vi "DCRI.vi"() -> ()   [LabVIEW 2024]
uses:
  EFmeter.lvlib
  <vilib>/Analysis/NI_AALBase.lvlib
  <vilib>/Analysis/baseanly.llb/Mean (DBL).vi
  BK Precision 8500B Series/BK Precision 8500B Series.lvlib
  <instrlib>/Zatez Kopper/Zatez Kopper.lvlib
panel:
  out "Aktualni zatez 2":dbl=2.5
  out "DCIR":dbl
  in  "Èas ustálení [ms]":dbl
  in  "LOAD":refnum<visa-resource-name>
  in  "Clear":bool
  in  "Typ zateze":u16(ring) items=["Manualni", "BK 8542B", "KOPPER-zatez"]
  in  "Ulozit data":bool
  in  "file path (use dialog)":path
  in  "Vzorku na krokù":u16 max=100 step=1
  in  "Prumerovani":bool
  in  "Zatezovaci proud [A]":dbl
  in  "EFmeter":refnum<visa-resource-name>
  in  "stop":bool
  in  "Start":bool
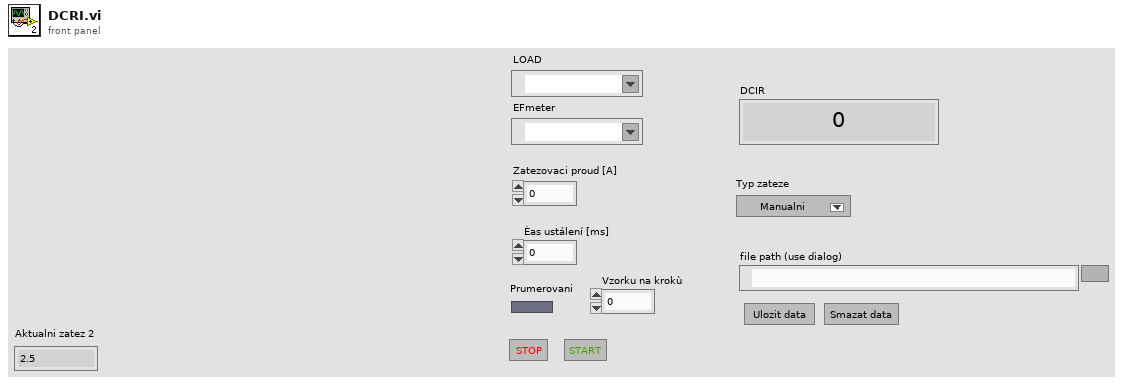
[diagram p1: front panel]
types:
  T1 = enum16{"init", "wait", "graph", "meas", "change_load", "init_measurment", "save", "clear"}
  T2 = enum16{"open", "replace", "create", "open or create", "replace or create", "replace or create with confirmation"}
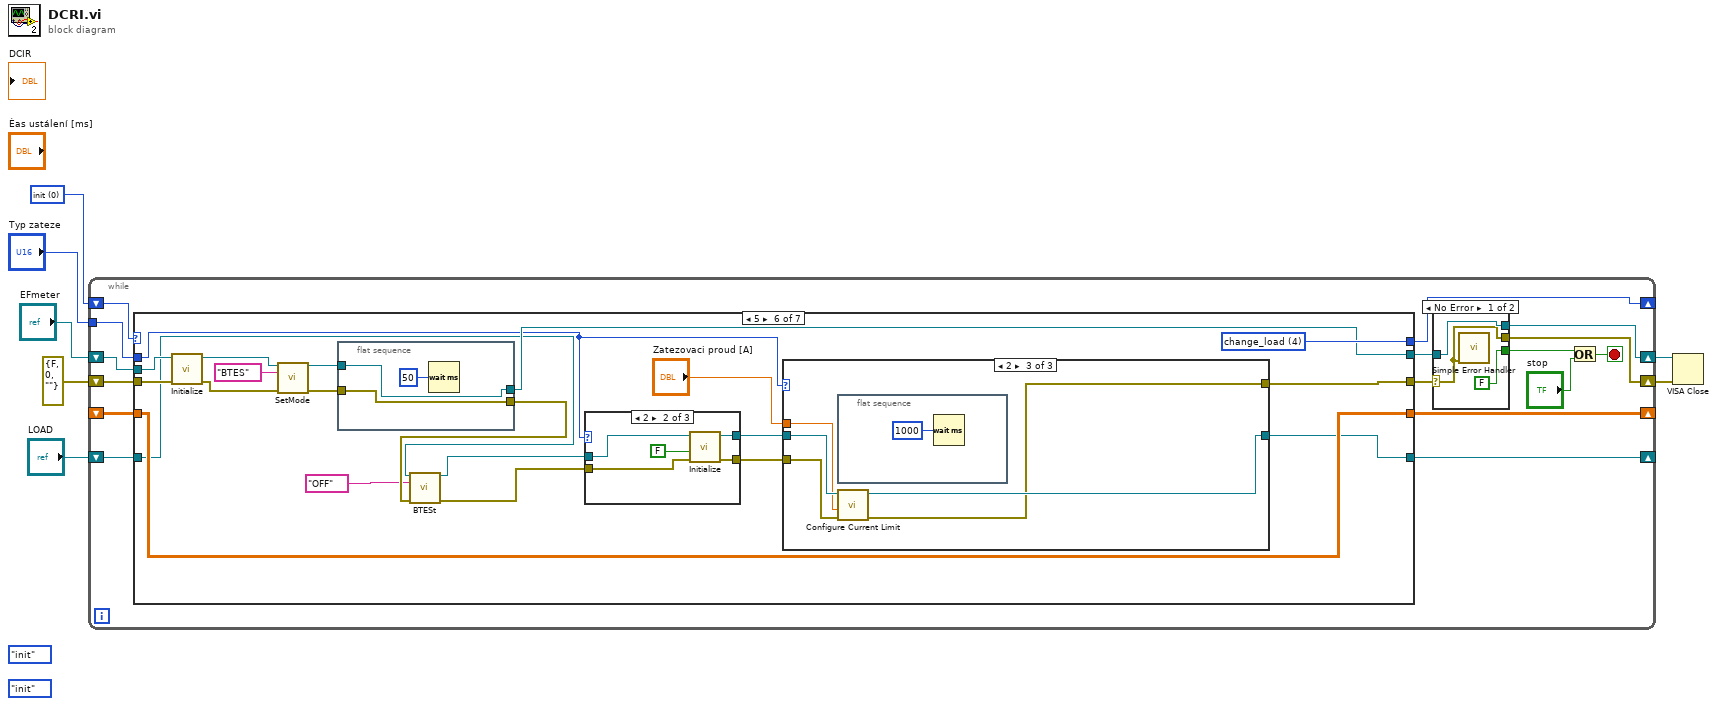
[diagram p0: block diagram]
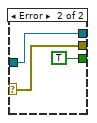
[diagram p2: hidden frame]
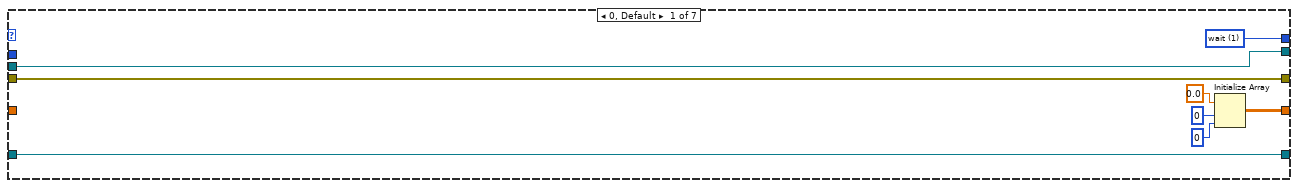
[diagram p3: hidden frame]
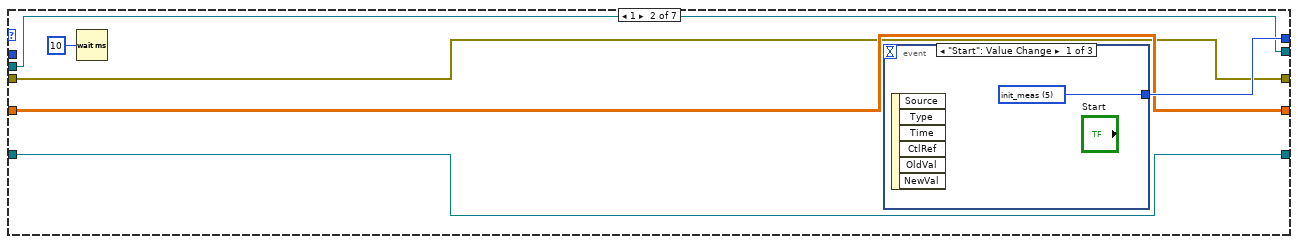
[diagram p4: hidden frame]
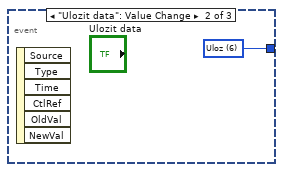
[diagram p5: hidden frame]
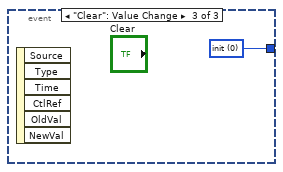
[diagram p6: hidden frame]
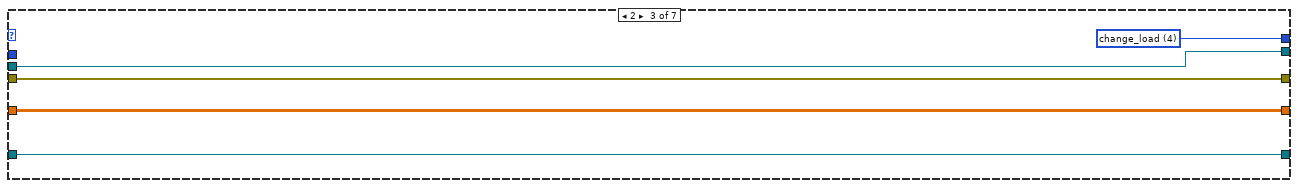
[diagram p7: hidden frame]
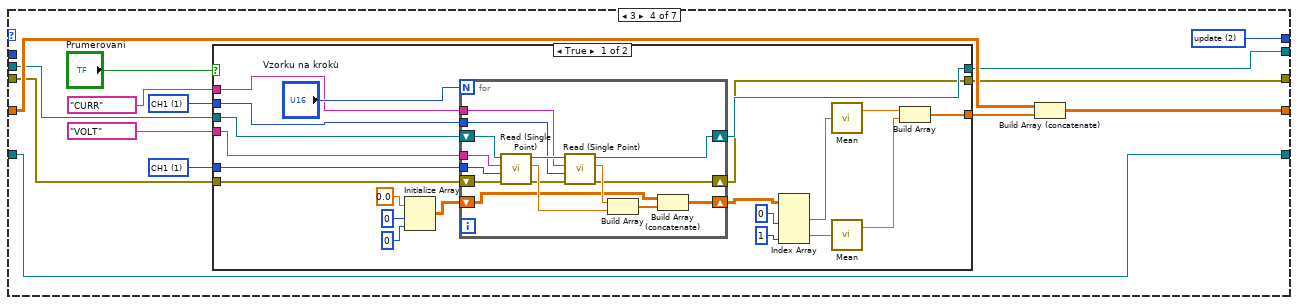
[diagram p8: hidden frame]
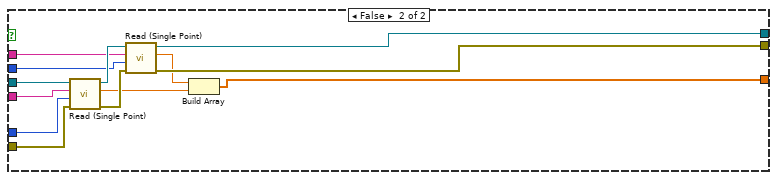
[diagram p9: hidden frame]
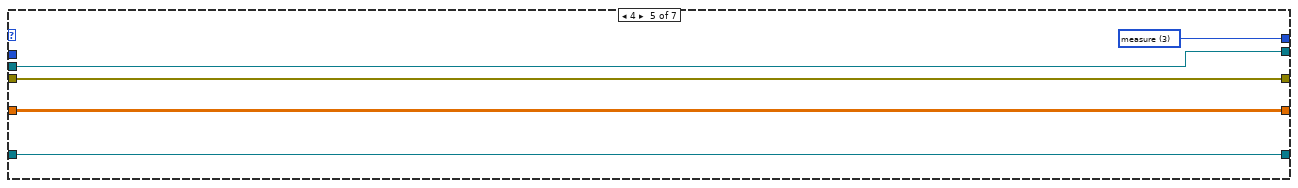
[diagram p10: hidden frame]
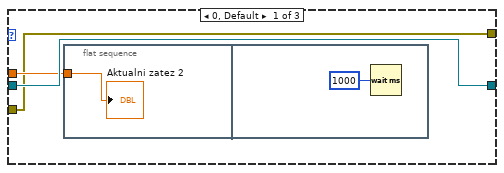
[diagram p11: hidden frame]
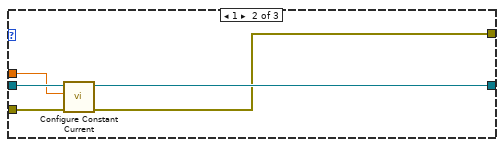
[diagram p12: hidden frame]
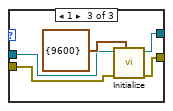
[diagram p14: hidden frame]
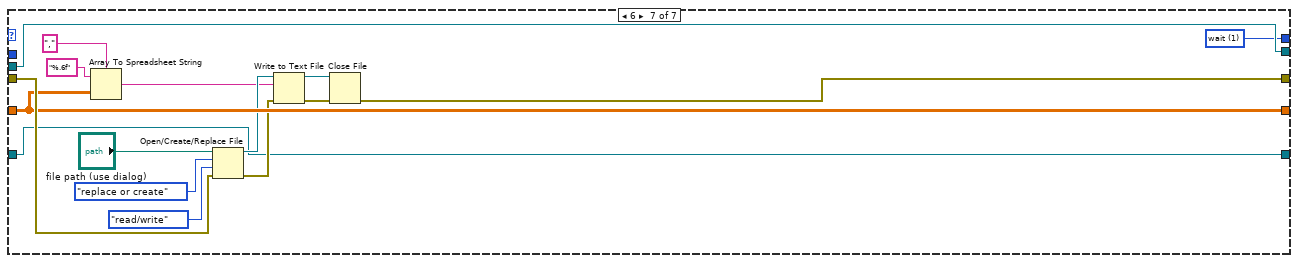
[diagram p15: hidden frame]
diagram:
  (unwired) T1."init"
  (unwired) T1."init"
  w7 = u16 0 items=["init", "wait", "update", "measure", "change_load", "init_meas", "Uloz", "clear"]
  n1 = while {
    shift-right: [w23] -> _
    shift-left: _ -> [w22]
    shift-right: [w18] -> _
    shift-left: w7 -> [w21]
    shift-right: [w15] -> w4
    shift-left: "EFmeter" -> [w20]
    shift-right: [w14] -> w3
    shift-left: errorcluster {"status"=FALSE, "code"=0, "source"=""} ("error in (no error)") -> [w19]
    tunnel: "Typ zateze" -> [w10]
    shift-right: [w9] -> _
    shift-left: "LOAD" -> [w8]
    stop <- w12 stop-if-true
    n2 = case shown="5" w21 {
      tunnel: [w35 w42 w51 w64 w119 w140 w182] -> w23
      tunnel: w22 -> [_ w42 w51 w65 w119 w140 w182]
      tunnel: [w34 w43 w47 w62 w115 w134 w180] -> w18
      tunnel: [w31 w40 w49 w54 w117 w128 w176] -> w17
      tunnel: [w32 w41 w50 w55 w116 w133 w187] -> w16
      tunnel: w20 -> [w32 w41 w50 w61 w116 w136 w187]
      tunnel: w19 -> [w31 w40 w49 w60 w117 w135 w183]
      tunnel: w10 -> [_ _ _ _ _ w125 _]
      tunnel: [w30 w38 w48 w52 w118 w127 w172] -> w9
      tunnel: w8 -> [w30 w38 w48 w52 w118 w124 w172]
      frame 0, Default {
        w34 = u16 1 items=["init", "wait", "update", "measure"]
        n3 = Initialize Array(0.0 ("element"), 0 ("dimension size"), 0 ("dimension size")) -> (w35:dbl[][])
      }
      frame 1 {
        n4 = Wait (ms)(milliseconds to wait=u32 10) -> ()  [unwired: 1 out]
        n5 = event shown="[0] \"Start\": Value Change" {
          selector: _ -> [_ _ _]
          dyn-events: _ -> [_ _ _]
          timeout: _ -> [_ _ _]
          tunnel: [w44 w45 w46] -> w43
          event "Start": Value Change {
            w44 = u16 5 items=["init", "wait", "update", "measure", "change_load", "init_meas"]
            n6 = event-data() -> ()  [unwired: 1 in, 6 out]
          }
          event "Ulozit data": Value Change {
            w45 = u16 6 items=["init", "wait", "update", "measure", "change_load", "init_meas", "Uloz"]
            n7 = event-data() -> ()  [unwired: 1 in, 6 out]
          }
          event "Clear": Value Change {
            w46 = u16 0 items=["init", "wait", "update", "measure", "change_load", "init_meas", "Uloz", "clear"]
            n8 = event-data() -> ()  [unwired: 1 in, 6 out]
          }
        }
      }
      frame 2 {
        w47 = u16 4 items=["init", "wait", "update", "measure", "change_load", "init_meas"]
      }
      frame 3 {
        w56 = u16 1 items=["CH2"=2, "CH1"=1] ("Ring")
        w59 = u16 1 items=["CH2"=2, "CH1"=1] ("Ring")
        w62 = u16 2 items=["init", "wait", "update", "measure"]
        n9 = case shown="True" "Prumerovani" {
          tunnel: [w68 w114] -> w63
          tunnel: w61 -> [w81 w113]
          tunnel: w60 -> [w80 w112]
          tunnel: w59 -> [w79 w111]
          tunnel: "VOLT" ("Combo Box") -> [w78 w110]
          tunnel: "CURR" ("Combo Box") -> [w77 w107]
          tunnel: w56 -> [w76 w106]
          tunnel: [w67 w105] -> w55
          tunnel: [w66 w104] -> w54
          frame True {
            n10 = Initialize Array(0.0 ("element"), 0 ("dimension size"), 0 ("dimension size")) -> (w82:dbl[][])
            n11 = for {
              N: "Vzorku na krokù" -> [_]
              shift-right: [w94] -> w67
              shift-left: w81 -> [w95]
              shift-right: [w92] -> w66
              shift-left: w80 -> [w93]
              tunnel: w79 -> [w91]
              tunnel: w78 -> [w90]
              tunnel: w77 -> [w89]
              tunnel: w76 -> [w88]
              shift-right: [w87] -> w75
              shift-left: w82 -> [w96]
              n12 = call "Read (Single Point).vi"("error in (no error)"=w93, "Ring"=w91, "Combo Box"=w90, "VISA resource name"=w95) -> ("error out"=w99:errorcluster, "Measurement"=w101:dbl, "VISA resource name out"=w100:refnum<visa-resource-name>)  [unwired: 5 in]
              n13 = call "Read (Single Point).vi"("error in (no error)"=w99, "Ring"=w88, "Combo Box"=w89, "VISA resource name"=w100) -> ("error out"=w92:errorcluster, "Measurement"=w98:dbl, "VISA resource name out"=w94:refnum<visa-resource-name>)  [unwired: 5 in]
              n14 = Build Array(w98, w101) -> (w97:dbl[])
              n15 = Build Array (concatenate)(w96, w97) -> (w87:dbl[][])
            }
            n16 = Index Array(array=w75, index (col) #1=0 ("disabled index (col)"), index (col) #2=1 ("index (col)")) -> (element #1=w74:dbl[], element #2=w73:dbl[])  [unwired: 2 in]
            n17 = call-poly <vilib>:"Mean.vi"("X"=w74) -> ("mean"=w70:dbl)  [unwired: 1 out]
            n18 = call-poly <vilib>:"Mean.vi"("X"=w73) -> ("mean"=w69:dbl)  [unwired: 1 out]
            n19 = Build Array(w70, w69) -> (w68:dbl[])
          }
          frame False {
            n20 = call "Read (Single Point).vi"("error in (no error)"=w112, "Ring"=w111, "Combo Box"=w110, "VISA resource name"=w113) -> ("error out"=w109:errorcluster, "Measurement"=w102:dbl, "VISA resource name out"=w108:refnum<visa-resource-name>)  [unwired: 5 in]
            n21 = call "Read (Single Point).vi"("error in (no error)"=w109, "Ring"=w106, "Combo Box"=w107, "VISA resource name"=w108) -> ("error out"=w104:errorcluster, "Measurement"=w103:dbl, "VISA resource name out"=w105:refnum<visa-resource-name>)  [unwired: 5 in]
            n22 = Build Array(w103, w102) -> (w114:dbl[])
          }
        }
        n23 = Build Array (concatenate)(w65, w63) -> (w64:dbl[][])
      }
      frame 4 {
        w115 = u16 3 items=["init", "wait", "update", "measure", "change_load", "init_meas", "Uloz", "clear"]
      }
      frame 5 {
        w134 = u16 4 items=["init", "wait", "update", "measure", "change_load", "init_meas"]
        n24 = call <instrlib>:"Initialize.vi"("error in (no error)"=w135, "VISA resource name"=w136) -> ("error out"=w139:errorcluster, "VISA resource name out"=w138:refnum<visa-resource-name>)  [unwired: 8 in]
        n25 = call "SetMode.vi"("VISA resource name"=w138, "Combo Box"="BTES", "error in (no error)"=w139) -> ("VISA resource name out"=w132:refnum<visa-resource-name>, "error out"=w131:errorcluster)  [unwired: 11 in]
        n26 = flat-sequence {
          tunnel: [w170] -> w133
          tunnel: w132 -> [w170]
          tunnel: w131 -> [w169]
          tunnel: [w169] -> w122
          frame #0 {
            n27 = Wait (ms)(milliseconds to wait=u32 50) -> ()  [unwired: 1 out]
          }
        }
        n28 = call "BTESt.vi"("VISA resource name"=w124, "Combo Box"="OFF", "error in (no error)"=w122) -> ("VISA resource name out"=w123:refnum<visa-resource-name>, "error out"=w121:errorcluster)  [unwired: 11 in]
        n29 = case shown="2" w125 {
          tunnel: w121 -> [w158 w162 w167]
          tunnel: [w158 w161 w166] -> w130
          tunnel: [w157 w160 w165] -> w129
          tunnel: w123 -> [w157 w163 w164]
          frame 0, Default {
          }
          frame 2 {
            n30 = call <instrlib>:"Initialize.vi"("error in (no error)"=w162, "Reset (True)"=FALSE, "VISA resource name"=w163) -> ("error out"=w161:errorcluster, "VISA resource name out"=w160:refnum<visa-resource-name>)  [unwired: 7 in]
          }
          frame 1 {
            n31 = call <instrlib>:"Initialize.vi"("Serial Configuration"=cluster{"Baud Rate":u32} {"Baud Rate"=9600}, "error in (no error)"=w167, "VISA resource name"=w164) -> ("error out"=w166:errorcluster, "VISA resource name out"=w165:refnum<visa-resource-name>)  [unwired: 7 in]
          }
        }
        n32 = case shown="2" w125 {
          tunnel: w129 -> [w143 w150 w152]
          tunnel: [w143 w149 w155] -> w127
          tunnel: "Zatezovaci proud [A]" -> [w142 w146 w151]
          tunnel: w130 -> [w141 w148 w153]
          tunnel: [w141 w147 w154] -> w128
          frame 0, Default {
            n33 = flat-sequence {
              tunnel: w142 -> [w144]
              frame #0 {
                "Aktualni zatez 2" <- w144
              }
              frame #1 {
                n34 = Wait (ms)(milliseconds to wait=u32 1000) -> ()  [unwired: 1 out]
              }
            }
          }
          frame 1 {
            n35 = call "Configure Constant Current.vi"("error in (no error)"=w148, "CC Current (0)"=w146, "VISA resource name"=w150) -> ("error out"=w147:errorcluster, "VISA resource name out"=w149:refnum<visa-resource-name>)  [unwired: 7 in]
          }
          frame 2 {
            n36 = flat-sequence {
              frame #0 {
                n37 = Wait (ms)(milliseconds to wait=u32 1000) -> ()  [unwired: 1 out]
              }
            }
            n38 = call <instrlib>:"Configure Current Limit.vi"("error in (no error)"=w153, "Current Limit (0.0 A)"=w151, "VISA resource name"=w152) -> ("error out"=w154:errorcluster, "VISA resource name out"=w155:refnum<visa-resource-name>)  [unwired: 7 in]
          }
        }
      }
      frame 6 {
        w180 = u16 1 items=["init", "wait", "update", "measure", "change_load", "init_meas"]
        n39 = Array To Spreadsheet String(delimiter (Tab)=",", array=w182, 3:"%.6f" ("format string")) -> (spreadsheet string=w173:string)
        n40 = Open/Create/Replace File(file path (use dialog)="file path (use dialog)", error in=w183, operation (0:open)=T2."replace or create", access (0:read/write)=enum16{"read/write", "read-only", "write-only"}."read/write") -> (refnum out=w175:refnum<file>, error out=w178:errorcluster)  [unwired: 2 in, 1 out]
        n41 = Write to Text File(file (use dialog)=w175, text=w173, error in=w178) -> (refnum out=w174:refnum<file>, error out=w177:errorcluster)  [unwired: 1 in, 1 out]
        n42 = Close File(refnum=w174, error in=w177) -> (error out=w176:errorcluster)  [unwired: 1 out]
      }
    }
    n43 = case shown="No Error" w17 {
      selector: w17 -> [w24 w28]
      tunnel: w16 -> [w26 w29]
      tunnel: [w26 w29] -> w15
      tunnel: [w24 w28] -> w14
      tunnel: [FALSE TRUE] -> w11
      frame No Error {
        n44 = call <vilib>:"Simple Error Handler.vi"("error in (no error)"=w24) -> ()  [unwired: 4 in, 5 out]
      }
      frame Error {
      }
    }
    n45 = Or(x=w11, y="stop") -> (x .or. y?=w12:bool)
  }
  n46 = VISA Close(VISA resource name=w4, error in (no error)=w3) -> ()  [unwired: 1 out]
